vi "mks946_set_voltage_full_scale.vi"(6 "err_in":errorcluster, 7 "visa_in":refnum<visa-resource-name>="COM3", 10 "channel":i32=1, 11 "address":i32=253) -> (0 "status":bool=TRUE, 2 "message":string, 3 "response":string, 4 "err_out":errorcluster={"status"=FALSE, "code"=1073676294, "source"="VISA Read in thcd_get_chan.vi"}, 5 "visa_out":refnum<visa-resource-name>="COM3")   [LabVIEW 2019]
panel:
  in  "full_scale":string
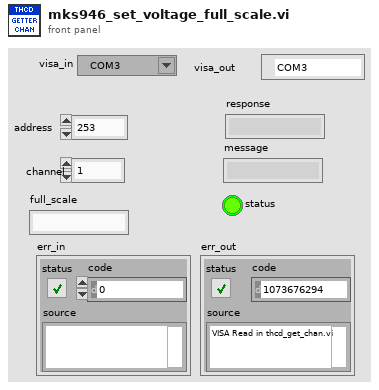
[diagram p1: front panel]
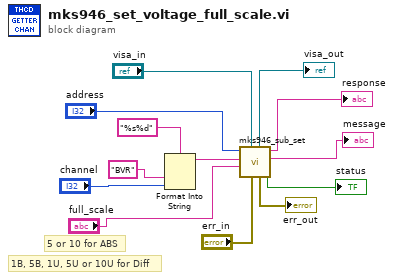
[diagram p0: block diagram]
diagram:
  # "1B, 5B, 1U, 5U or 10U for Diff"
  # "5 or 10 for ABS"
  n1 = Format Into String(format string="%s%d", "BVR" ("mks946_comm"), "channel") -> (resulting string=w4:string)  [unwired: 2 in, 1 out]
  n2 = call "mks946_sub_set.vi"("error in (no error)"="err_in", "VISA_ref_in"="visa_in", "parameter"="full_scale", "command"=w4, "address"="address") -> ("status"=→"status":bool, "message"=→"message":string, "response"=→"response":string, "error out"=→"err_out":errorcluster, "VISA_ref_out"=→"visa_out":refnum<visa-resource-name>)  [unwired: 2 in]
